vi "FlatToRichnixnet_grpc_DbCloseDatabaseResponse.vi"(5 "OutputClusterType":T1, 11 "InputCluster":T2) -> (3 "OutputCluster":T1)   [LabVIEW 2025, in "xnet-grpc_client.lvlib"]
uses:
  xnet-grpc_client.lvlib
  nixnet_grpc_DbCloseDatabaseResponse_Flat.ctl
  nixnet_grpc_DbCloseDatabaseResponse.ctl
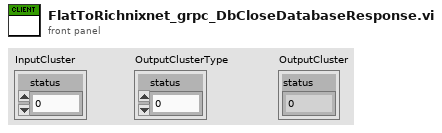
[diagram p1: front panel]
types:
  T1 = typedef "xnet-grpc_client.lvlib/nixnet_grpc_DbCloseDatabaseResponse.ctl" = cluster{"status":i32}
  T2 = typedef "xnet-grpc_client.lvlib/nixnet_grpc_DbCloseDatabaseResponse_Flat.ctl" = cluster{"status":i32}
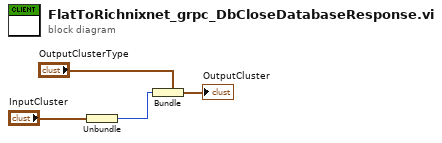
[diagram p0: block diagram]
diagram:
  n1 = Unbundle "Unbundle"("InputCluster") -> ("status"=w1:i32)
  n2 = Bundle "Bundle"(cluster="OutputClusterType", "status"=w1) -> (→"OutputCluster":T1)
